vi "Load Virtual Instruments.vi"(8 "Error In":errorcluster, 10 "Source":string) -> (0 "Error Out":errorcluster)   [LabVIEW 2024, in "Instrument Manager.lvclass"]
uses:
  Instrument Manager.lvclass
  Config from JSON/Config from JSON.lvclass
  03154150-9636-41b2-8ac1-c8a1f310a941.vi
  03154150-9636-41b2-8ac1-c8a1f310a941.vi/a4169a97-72fc-4003-a778-603cf20cafa0.vi
  <vilib>/Utility/error.llb/Trim Whitespace.vi
  <vilib>/JDP Science/JSONtext/Find Item.vi
  <vilib>/Utility/error.llb/Trim Whitespace One-Sided.vi
  <vilib>/JDP Science/JSONtext/Next JSON Value.vi
  <vilib>/JDP Science/JSONtext/String Subset.vi
  <vilib>/JDP Science/JSONtext/Parsing/Advance past next JSON Value (inlined COPY).vi
  <vilib>/JDP Science/JSONtext/Parsing/Advance past whitespace.vi
  <vilib>/JDP Science/JSONtext/Parsing/Advance past String.vi
  <vilib>/JDP Science/JSONtext/Parsing/Advance past Number.vi
  <vilib>/JDP Science/JSONtext/Parsing/Advance past Line Ending.vi
  <vilib>/JDP Science/JSONtext/Parsing/Parse Full Path or Item Name.vi
  <vilib>/JDP Science/JSONtext/Parsing/Advance past Array.vi
  <vilib>/JDP Science/JSONtext/Parsing/Advance past Object.vi
  <vilib>/JDP Science/JSONtext/support/Error Cluster From Code.vi
  <vilib>/JDP Science/JSONtext/Offset/Find Item Locations by Path.vi
  <vilib>/JDP Science/JSONtext/JSON text to Variant.vi
  Common-LabVIEW-Helpers/Source/errors/-8301 Item not found in JSON--error.vi
  Common-LabVIEW-Helpers/Source/errors/-8300 JSON empty--error.vi
  <vilib>/JDP Science/JSONtext/LVClass Serializer/JSONtext LVClass Serializer.lvclass
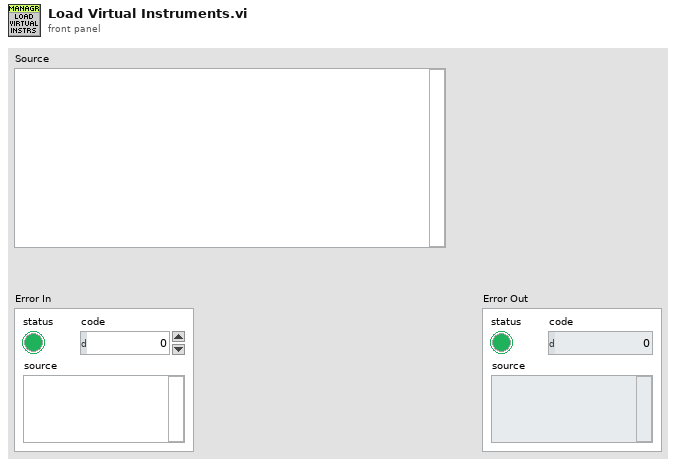
[diagram p1: front panel]
types:
  T1 = typedef "Instrument Manager.lvclass/ObjectAttributes.ctl" = cluster{"IInstruments":map{string, refnum<class "IInstrument.lvclass">}, "IVirtual Instruments":map{string, refnum<class "IVirtual Instrument.lvclass">}, "Instrument Configurations":map{string, refnum<class "Config from JSON.lvclass">}, "Virtual Instrument Configurations":map{string, refnum<class "Config from JSON.lvclass">}, "Action Point Configurations":map{string, refnum<class "Config from JSON.lvclass">}, "Action Points":map{string, refnum<class "Action Point.lvclass">}}
  T2 = map{string, refnum<class "Config from JSON.lvclass">}
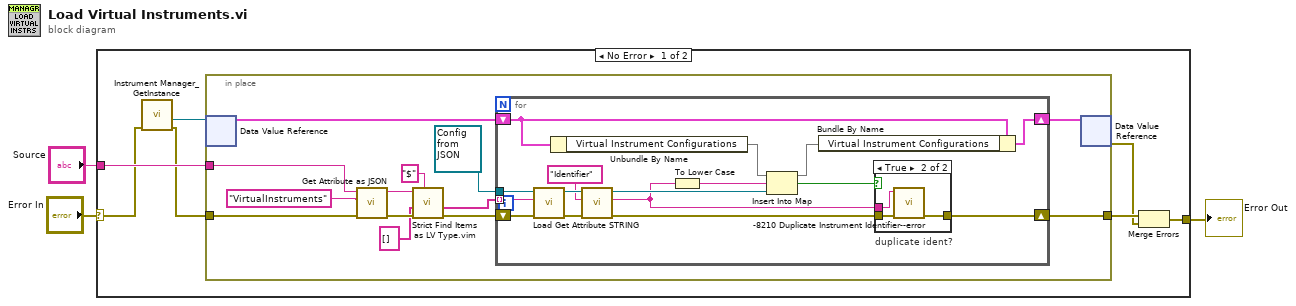
[diagram p0: block diagram]
diagram:
  n1 = case shown="No Error" "Error In" {
    selector: "Error In" -> [w9 w44]
    tunnel: [w5 w44] -> w3
    tunnel: "Source" -> [w10 _]
    frame No Error {
      n2 = call "Instrument Manager_GetInstance.vi"("Error In"=w9) -> ("Error Out"=w8:errorcluster, "DVRRefOut"=w6:refnum<data-value>)  [unwired: 6 in, 3 out]
      n3 = in-place {
        in-place-border: w10 -> [w18]
        in-place-border: w8 -> [w23]
        in-place-border: [w20] -> w7
        n4 = in-place-dvr #1(w6) -> (w21:T1)  [unwired: 1 out]
        n5 = call "Get Attribute as JSON.vi"("error in"=w23, "Attribute"="VirtualInstruments", "Source"=w18) -> ("error out"=w22:errorcluster, "<JSON>"=w17:string)  [unwired: 7 in]
        n6 = call "Strict Find Items as LV Type.vim"("$Path or Item Name"="$", "error in"=w22, "Data Type and Default Value"=string[] [], "<JSON>"=w17) -> ("error out"=w14:errorcluster, "Data out"=w13:string[])  [unwired: 5 in, 1 out]
        n7 = for {
          shift-right: [w37] -> w20
          shift-left: w14 -> [w39]
          tunnel: w13 -> [w34] mode=indexing
          shift-right: [w35] -> w19
          shift-left: w21 -> [w36]
          tunnel: refnum<class "Config from JSON.lvclass"> refnum ("Config From JSON in") -> [w33]
          n8 = call-dynamic "Load.vi"("error in"=w39, "Source"=w34, "Config From JSON in"=w33) -> ("error out"=w38:errorcluster, "Config From JSON out"=w32:refnum<class "Config from JSON.lvclass">)  [unwired: 7 in]
          n9 = Unbundle By Name(w36) -> ("Virtual Instrument Configurations"=w30:T2)
          n10 = call-dynamic "Get Attribute STRING.vi"("error in"=w38, "Attribute"="Identifier" ("$Path or Item Name"), "ConfigFromJSON in"=w32) -> ("error out"=w24:errorcluster, "Value"=w25:string, "ConfigFromJSON out"=w28:refnum<class "Config from JSON.lvclass">)  [unwired: 6 in]
          n11 = To Lower Case(string=w25) -> (all lower case string=w26:string)
          n12 = Insert Into Map(map in=w30, key=w26, value=w28) -> (map out=w27:T2, key already included?=w29:bool)  [unwired: 1 out]
          n13 = Bundle By Name(cluster=w36, "Virtual Instrument Configurations"=w27) -> (w35:T1)
          n14 = case "duplicate ident?" shown="True" w29 {
            tunnel: w24 -> [w40 w43]
            tunnel: [w40 w42] -> w37
            tunnel: w25 -> [_ w41]
            frame False {
            }
            frame True {
              n15 = call "-8210 Duplicate Instrument Identifier--error.vi"("error in"=w43, "Instrument Identifier"=w41) -> ("error out"=w42:errorcluster)  [unwired: 9 in]
            }
          }
        }
        n16 = in-place-dvr #1(w19) -> (w4:errorcluster)  [unwired: 1 out]
      }
      n17 = Merge Errors(w7, w4) -> (w5:errorcluster)
    }
    frame Error {
    }
  }
  "Error Out" <- w3
